vi "Polyphase Filter (1D, CSG).vi"(6 "zero phase? (T)":bool=TRUE, 7 "init? (F)":bool, 8 "error in (no error)":errorcluster, 9 "factor":T1={"interpolation"=1, "decimation"=1}, 10 "FIR Coefficients":sgl[](array[numeric]), 11 "X":csg[](array[numeric])) -> (0 "error out":errorcluster, 3 "Filtered X":csg[](array[numeric]))   [LabVIEW 2020, in "NI_AAL_Filter.lvlib"]
doc: "Filters a signal continuously with a multirate filter."
uses:
  <vilib>/Analysis/NI_AAL_Filter.lvlib
  <vilib>/Analysis/3filter.llb/Polyphase Filter_Factor.ctl
  <vilib>/Analysis/NI_AALPro.lvlib
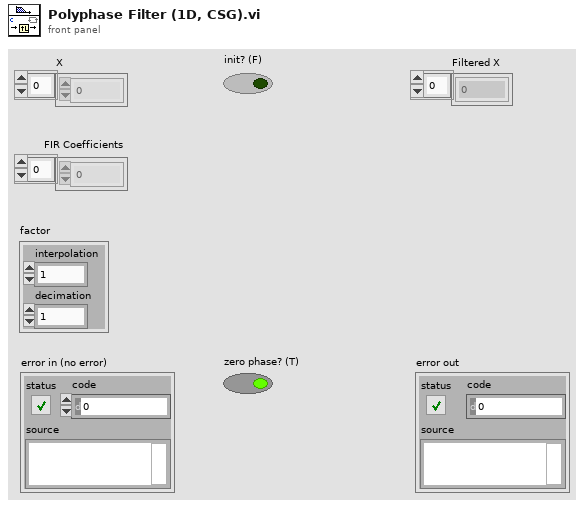
[diagram p1: front panel]
types:
  T1 = typedef "NI_AAL_Filter.lvlib/Polyphase Filter_Factor.ctl" = cluster{"interpolation":i32, "decimation":i32}
  T2 = typedef "NI_AAL_Filter.lvlib/Polyphase Filter_Mode.ctl" = i32
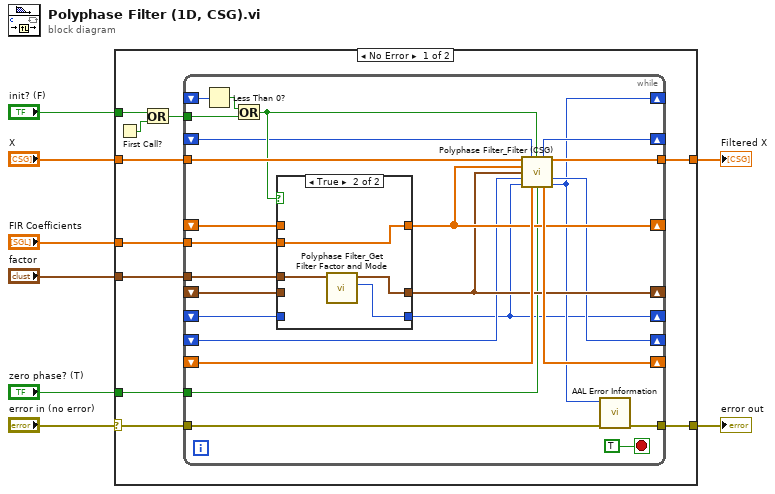
[diagram p0: block diagram]
diagram:
  n1 = case shown="No Error" "error in (no error)" {
    selector: "error in (no error)" -> [w17 w51]
    tunnel: "factor" -> [w18 _]
    tunnel: "FIR Coefficients" -> [w16 _]
    tunnel: "X" -> [w15 _]
    tunnel: [w10 w51] -> w2
    tunnel: "init? (F)" -> [w13 _]
    tunnel: [w11 _] -> w4
    tunnel: "zero phase? (T)" -> [w9 _]
    frame No Error {
      n2 = First Call?() -> (First Call?: T/F=w14:bool)
      n3 = Or(x=w13, y=w14) -> (x .or. y?=w12:bool)
      n4 = while {
        tunnel: w18 -> [w41]
        tunnel: w16 -> [w42]
        tunnel: w15 -> [w40]
        tunnel: w12 -> [w27]
        shift-right: [w22] -> _
        shift-left: _ -> [w23]
        shift-right: [w21] -> _
        shift-left: _ -> [w20]
        shift-right: [w38] -> _
        shift-left: _ -> [w39]
        tunnel: [w37] -> w11
        shift-right: [w34] -> _
        shift-left: _ -> [w31]
        shift-right: [w32] -> _
        shift-left: _ -> [w33]
        shift-right: [w19] -> _
        shift-left: _ -> [w30]
        tunnel: w9 -> [w28]
        shift-right: [w24] -> _
        shift-left: _ -> [w25]
        tunnel: w17 -> [w36]
        tunnel: [w35] -> w10
        stop <- TRUE stop-if-true
        n5 = Less Than 0?(x=w20) -> (x < 0?=w26:bool)
        n6 = Or(x=w26, y=w27) -> (x .or. y?=w29:bool)
        n7 = case shown="True" w29 {
          tunnel: w41 -> [_ w50]
          tunnel: [w45 w49] -> w34
          tunnel: w42 -> [_ w49]
          tunnel: [w46 w48] -> w32
          tunnel: w33 -> [w46 _]
          tunnel: w31 -> [w45 _]
          tunnel: [w44 w47] -> w19
          tunnel: w30 -> [w44 _]
          frame False {
          }
          frame True {
            n8 = call <vilib>:"Polyphase Filter_Get Filter Factor and Mode.vi"("factor in"=w50) -> ("mode"=w47:T2, "factor out"=w48:T1)  [unwired: 9 in]
          }
        }
        n9 = call <vilib>:"Polyphase Filter_Filter (CSG).vi"("X"=w40, "output phase in"=w25, "init? (F)"=w29, "FIR Coefficients"=w34, "factor"=w32, "skip point in"=w23, "mode"=w19, "State in"=w39, "zero phase? (T)"=w28) -> ("output phase out"=w24:i32, "Filtered X"=w37:csg[], "skip point out"=w22:i32, "State out"=w38:csg[], "error"=w21:i32)  [unwired: 2 in]
        n10 = call <vilib>:"AAL Error Information.vi"("error in (no error)"=w36, "error code"=w21) -> ("error out"=w35:errorcluster)  [unwired: 9 in]
      }
    }
    frame Error {
    }
  }
  "Filtered X" <- w4
  "error out" <- w2
